vi "Create Known Type.vi"(10 "Name":string, 11 "Type":refnum<class>) -> (3 "Known Type":T1)   [LabVIEW 2017, in "Known Types Binder.lvclass"]
uses:
  Known Types Binder.lvclass
  Known Type.ctl
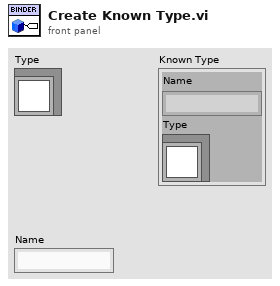
[diagram p1: front panel]
types:
  T1 = typedef "Known Types Binder.lvclass/Known Type.ctl" = cluster{"Name":string, "Type":refnum<class>}
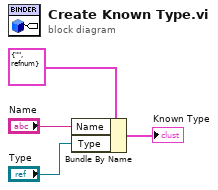
[diagram p0: block diagram]
diagram:
  n1 = Bundle By Name(cluster=T1 {"Name"="", "Type"=refnum} ("Known Type"), "Name"="Name", "Type"="Type") -> (→"Known Type":T1)
